vi "FP_Find Point on Window.vi"(8 "Error":errorcluster, 9 "Position":T1, 11 "Window":T2) -> (0 "Error Out":errorcluster, 3 "Point Out":T3)   [LabVIEW 2015]
uses:
  TypeDefs_Utility/Cluster_Top Left position.ctl
  <vilib>/Utility/miscctls.llb/LVRectTypeDef.ctl
  TypeDefs_Utility/ENUM RB_Pos_Quadrant Position.ctl
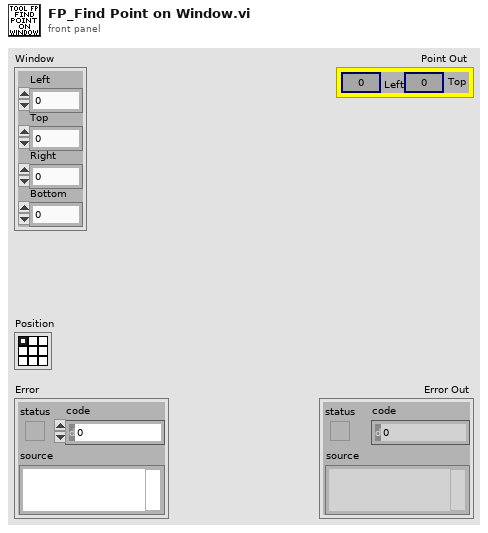
[diagram p1: front panel]
types:
  T1 = typedef "ENUM RB_Pos_Quadrant Position.ctl" = enum32{"LFT-TOP", "MID-TOP", "RGT-TOP", "LFT-CTR", "MID-CTR", "RGT-CTR", "LFT-BOT", "MID-BOT", "RGT-BOT"}
  T2 = typedef "LVRectTypeDef.ctl" = cluster{"Left":i16, "Top":i16, "Right":i16, "Bottom":i16}
  T3 = typedef "Cluster_Top Left position.ctl" = cluster{"Left":i32, "Top":i32}
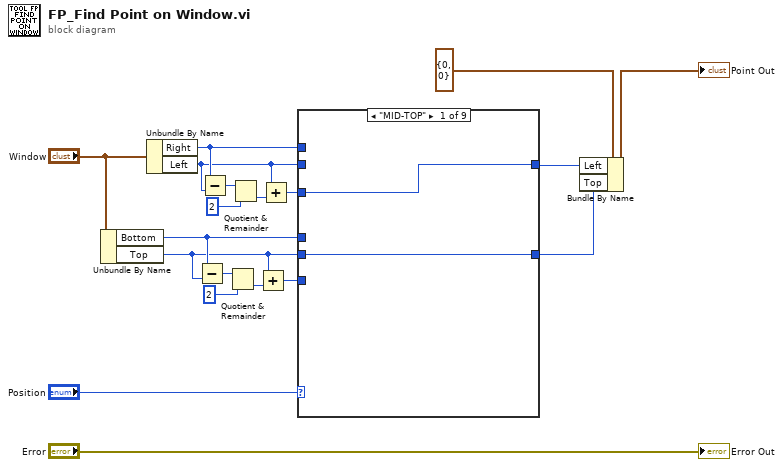
[diagram p0: block diagram]
diagram:
  n1 = Unbundle By Name("Window") -> ("Bottom"=w5:i16, "Top"=w3:i16)
  n2 = Unbundle By Name("Window") -> ("Right"=w14:i16, "Left"=w11:i16)
  n3 = Subtract(x=w5, y=w3) -> (x-y=w8:i16)
  n4 = Subtract(x=w14, y=w11) -> (x-y=w13:i16)
  n5 = Quotient & Remainder(x=w8, y=i16 2) -> (floor(x/y)=w7:i16)  [unwired: 1 out]
  n6 = Quotient & Remainder(x=w13, y=i16 2) -> (floor(x/y)=w12:i16)  [unwired: 1 out]
  n7 = Add(x=w3, y=w7) -> (x+y=w4:i16)
  n8 = Add(x=w11, y=w12) -> (x+y=w9:i16)
  n9 = case shown="\"MID-TOP\"" "Position" {
    tunnel: w14 -> [_ w23 _ _ w29 _ _ w35 _]
    tunnel: w11 -> [_ _ w25 _ _ w31 _ _ w37]
    tunnel: w9 -> [w21 _ _ w27 _ _ w33 _ _]
    tunnel: w5 -> [_ _ _ _ _ w30 w32 w34 _]
    tunnel: w3 -> [w20 w22 _ _ _ _ _ _ w36]
    tunnel: w4 -> [_ _ w24 w26 w28 _ _ _ _]
    tunnel: [w21 w23 w25 w27 w29 w31 w33 w35 w37] -> w2
    tunnel: [w20 w22 w24 w26 w28 w30 w32 w34 w36] -> w1
    frame "MID-TOP" {
    }
    frame "RGT-TOP" {
    }
    frame "LFT-CTR" {
    }
    frame "MID-CTR" {
    }
    frame "RGT-CTR" {
    }
    frame "LFT-BOT" {
    }
    frame "MID-BOT" {
    }
    frame "RGT-BOT" {
    }
    frame "LFT-TOP" {
    }
  }
  n10 = Bundle By Name(cluster=T3 {"Left"=0, "Top"=0} ("Point Out"), "Left"=w2, "Top"=w1) -> (→"Point Out":T3)
  "Error Out" <- "Error"
